vi "Single Questionable Register Condition Query.vi"(8 "error in":errorcluster, 11 "Instrument Handle In":i32) -> (0 "error out":errorcluster, 2 "Questionable Register":i32 format="%.0x", 3 "Instrument Handle Out":i32)   [LabVIEW 8.6, in "ZTScopeM.lvlib"]
doc: "Query the present condition of the questionable status register."
uses:
  ZTScopeM.lvlib
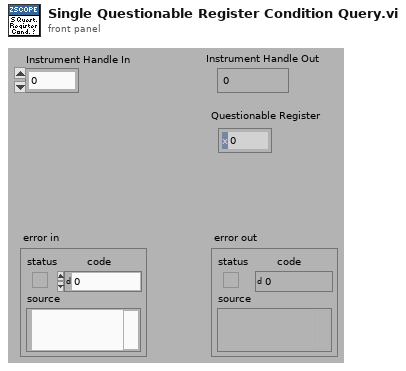
[diagram p1: front panel]
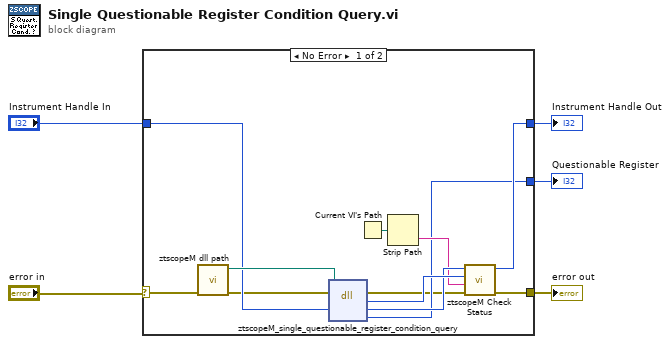
[diagram p0: block diagram]
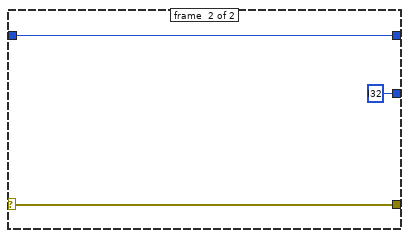
[diagram p2: hidden frame]
diagram:
  n1 = case shown="No Error" "error in" {
    selector: "error in" -> [w10 w20]
    tunnel: [w12 w20] -> w4
    tunnel: [w13 w18] -> w3
    tunnel: [w11 i32 ? ("enable")] -> w2
    tunnel: "Instrument Handle In" -> [w8 w18]
    frame #0 {
      n2 = call "ztscopeM dll path.vi"("error in (no error)"=w10) -> ("error out"=w7:errorcluster, "<instrument>.dll path"=w9:path)  [unwired: 9 in]
      n3 = dll-call lib="C:/Program Files (x86)/National Instruments/LabVIEW 2013/instr.lib/ztscopem/ztscopeM.dll" fn="ztscopeM_single_questionable_register_condition_query"(path in=w9, error in=w7, "instrumentHandle"=w8) -> (error out=w6:errorcluster, w17:i32, "instrumentHandle"=w16:i32, "questionableRegister"=w11:i32)  [unwired: 1 in, 2 out]
      n4 = Current VI's Path() -> (path=w15:path)
      n5 = Strip Path(path=w15) -> (name=w14:string)  [unwired: 1 out]
      n6 = call "ztscopeM Check Status.vi"("error in"=w6, "name of VI"=w14, "status (return code)"=w17, "instrument handle in"=w16) -> ("error out"=w12:errorcluster, "instrument handle out"=w13:i32)  [unwired: 2 out]
    }
    frame #1 {
    }
  }
  "Instrument Handle Out" <- w3
  "error out" <- w4
  "Questionable Register" <- w2
